vi "Ctor.vi"(8 "error in (no error)":errorcluster) -> (0 "error out":errorcluster, 3 "TargetPluginManager out":refnum<class "PlatformPluginManager.lvclass">)   [LabVIEW 2020, in "PicoG-Core.lvlib" / "PlatformPluginManager.lvclass"]
uses:
  PlatformPluginManager.lvclass
  Ref Data.ctl
  DeployPlatform/DeployPlatform.lvclass
  DeployResource/DeployResource.lvclass
  PlatformPluginManager.lvclass/PlatformPluginManager.ctl
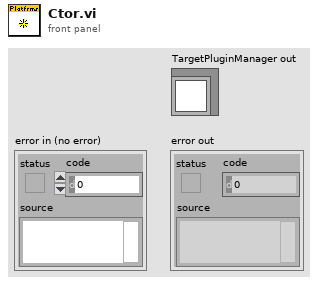
[diagram p1: front panel]
types:
  T1 = typedef "PicoG-Core.lvlib/PlatformPluginManager.lvclass/Ref Data.ctl" = cluster{"Platforms":refnum<class "DeployPlatform.lvclass">[], "Last Platform":refnum<class "DeployPlatform.lvclass">, "Last Resource":refnum<class "DeployResource.lvclass">}
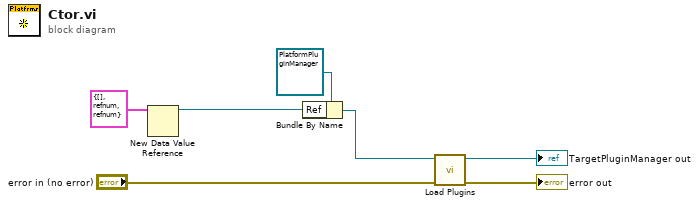
[diagram p0: block diagram]
diagram:
  n1 = New Data Value Reference(data value=T1 {"Platforms"=[], "Last Platform"=refnum, "Last Resource"=refnum} ("Ref Data")) -> (data value reference=w5:refnum<data-value>)  [unwired: 1 in, 1 out]
  n2 = Bundle By Name(cluster=refnum<class "PlatformPluginManager.lvclass"> refnum ("TargetPluginManager in"), "Ref"=w5) -> (w2:refnum<class "PlatformPluginManager.lvclass">)
  n3 = call "Load Plugins.vi"("error in (no error)"="error in (no error)", "TargetPluginManager in"=w2) -> ("error out"=→"error out":errorcluster, "TargetPluginManager out"=→"TargetPluginManager out":refnum<class "PlatformPluginManager.lvclass">)  [unwired: 8 in]
